vi "dvp Vi Get Input Io Level.vi"(9 "pInputIoLevel":bool, 10 "inputIo":u32(ring)=32769 items=["INPUT_IO_1"=32769, "INPUT_IO_2"=32770, "INPUT_IO_3"=32771, "INPUT_IO_4"=32772, "INPUT_IO_5"=32773, "INPUT_IO_6"=32774, "INPUT_IO_7"=32775, "INPUT_IO_8"=32776], 11 "handle":u32) -> (1 "pInputIoLevel out":bool, 3 "function return":u32(ring))   [LabVIEW 2018, in "LabViewDVPCamera.lvlib"]
doc: "LabviewDvp2Api dvpStatus dvpViGetInputIoLevel(dvpHandle handle, dvpInputIo inputIo, bool *pInputIoLevel);"
uses:
  LabViewDVPCamera.lvlib
  LabViewDVPCamera/LabViewDVPCamera.dll
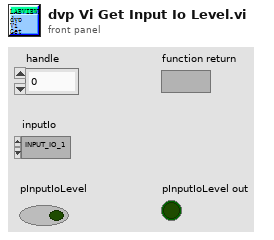
[diagram p1: front panel]
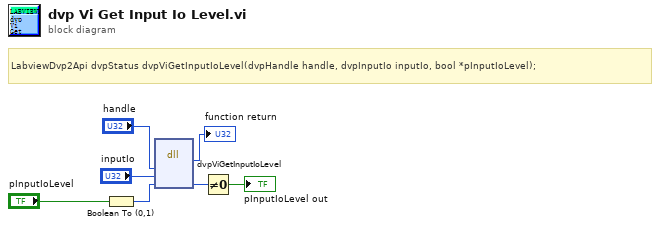
[diagram p0: block diagram]
diagram:
  # "LabviewDvp2Api dvpStatus dvpViGetInputIoLevel(dvpHandle handle, dvpInputIo inputIo, bool *pInputIoLevel);"
  n1 = Boolean To (0,1)(Boolean="pInputIoLevel") -> (0, 1=w3:i16)
  n2 = dll-call lib="C:/Program Files (x86)/DVP2 Labview cn 64/Sample/LabViewDVPCamera/LabViewDVPCamera.*" fn="dvpViGetInputIoLevel"("handle"="handle", "inputIo"="inputIo", "pInputIoLevel"=w3) -> (→"function return":u32, "pInputIoLevel"=w1:u8)  [unwired: 5 in, 2 out]
  n3 = Not Equal To 0?(x=w1) -> (x != 0?=→"pInputIoLevel out":bool)
